vi "Apply.vi"(8 "Error In":errorcluster, 11 "object in":refnum<class "Fetch Display CFG.lvclass">) -> (0 "Error Out":errorcluster, 3 "object out":refnum<class "Fetch Display CFG.lvclass">)   [LabVIEW 2023, in "OWON SDS1022.lvlib" / "Fetch Display CFG.lvclass"]
uses:
  Fetch Display CFG.lvclass
  Fetch Display CFG.lvclass/Fetch Display CFG.ctl
  SDS1000 Base CFG/SDS1000 Base CFG.lvclass
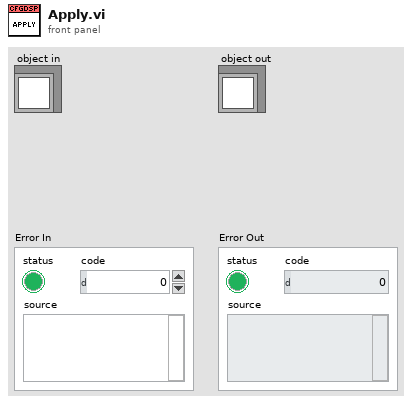
[diagram p1: front panel]
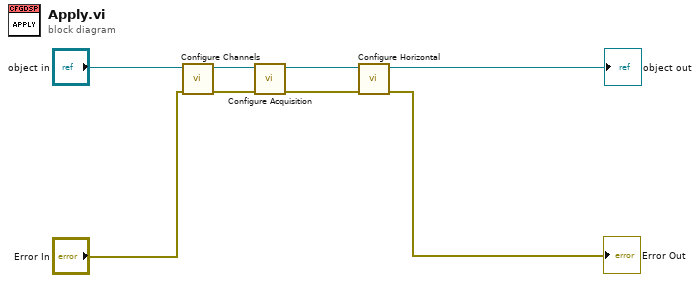
[diagram p0: block diagram]
diagram:
  n1 = call-dynamic "Configure Channels.vi"("error in"="Error In", "object in"="object in") -> ("error out"=w6:errorcluster, "object out"=w4:refnum<class "Fetch Display CFG.lvclass">)  [unwired: 8 in]
  n2 = call-dynamic "Configure Acquisition.vi"("error in"=w6, "Continuous Waveform Acq CFG in"=w4) -> ("error out"=w5:errorcluster, "Continuous Waveform Acq CFG out"=w2:refnum<class "Fetch Display CFG.lvclass">)  [unwired: 8 in]
  n3 = call "Configure Horizontal.vi"("error in (no error)"=w5, "object in"=w2) -> ("error out"=→"Error Out":errorcluster, "object out"=→"object out":refnum<class "Fetch Display CFG.lvclass">)  [unwired: 8 in]
